vi "Set Auto Logoff.vi"(8 "error in (no error)":errorcluster, 10 "Timer.AutoLogoff":dbl, 11 "Master in":refnum<class "Master.lvclass">) -> (0 "error out":errorcluster, 3 "Master out":refnum<class "Master.lvclass">)   [LabVIEW 2014, in "Master.lvclass"]
uses:
  Master/Master.lvclass
  Master/Master.lvclass/Master.ctl
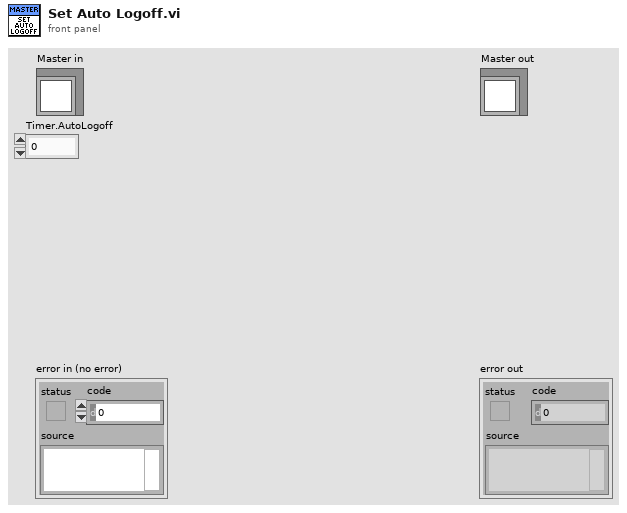
[diagram p1: front panel]
types:
  T1 = cluster{"Admin Password":string, "AutoLogoff":dbl}
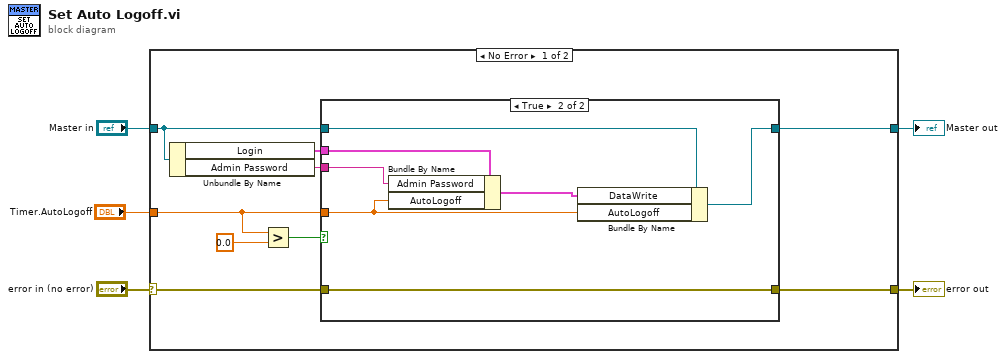
[diagram p0: block diagram]
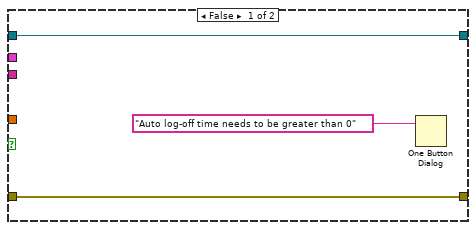
[diagram p2: hidden frame]
diagram:
  n1 = case shown="No Error" "error in (no error)" {
    selector: "error in (no error)" -> [w13 w26]
    tunnel: [w12 w26] -> w4
    tunnel: [w14 w25] -> w2
    tunnel: "Master in" -> [w8 w25]
    tunnel: "Timer.AutoLogoff" -> [w11 _]
    frame No Error {
      n2 = Unbundle By Name(w8) -> ("Login"=w7:T1, "Admin Password"=w6:string)
      n3 = Greater?(x=w11, y=0.0) -> (0:w9:bool)
      n4 = case shown="True" w9 {
        tunnel: w8 -> [w17 w24]
        tunnel: [w17 w23] -> w14
        tunnel: w11 -> [_ w20]
        tunnel: w13 -> [w16 w22]
        tunnel: [w16 w22] -> w12
        tunnel: w7 -> [_ w21]
        tunnel: w6 -> [_ w18]
        frame False {
          n5 = One Button Dialog(message="Auto log-off time needs to be greater than 0") -> ()  [unwired: 1 in, 1 out]
        }
        frame True {
          n6 = Bundle By Name(cluster=w21, "Admin Password"=w18, "AutoLogoff"=w20) -> (w19:T1)
          n7 = Bundle By Name(cluster=w24, "DataWrite"=w19, "AutoLogoff"=w20) -> (w23:refnum<class "Master.lvclass">)
        }
      }
    }
    frame Error {
    }
  }
  "error out" <- w4
  "Master out" <- w2
